vi "DAQmx for CI and AI.vi"() -> (2 "CI Timing Setting":T1={"Sample Clock Source"="PFI0", "Sample Rate"=5.0, "Samples per Loop"=1}, 3 "CI Channel Setting":T2={"Counter"="Dev1/ctr0", "A Input Terminal"="PFI8", "B Input Terminal"="PFI10", "Pulses Per Revolution"=24, "Z Index Enable"=FALSE, "Z Index Terminal"="PFI9"})   [LabVIEW 2017]
panel:
  in  "Timing Setting":T1={"Sample Clock Source"="PFI0", "Sample Rate"=5.0, "Samples per Loop"=1}
  in  "Channel Setting":T2={"Counter"="Dev1/ctr0", "A Input Terminal"="PFI8", "B Input Terminal"="PFI10", "Pulses Per Revolution"=24, "Z Index Enable"=FALSE, "Z Index Terminal"="PFI9"}
  # "CI"
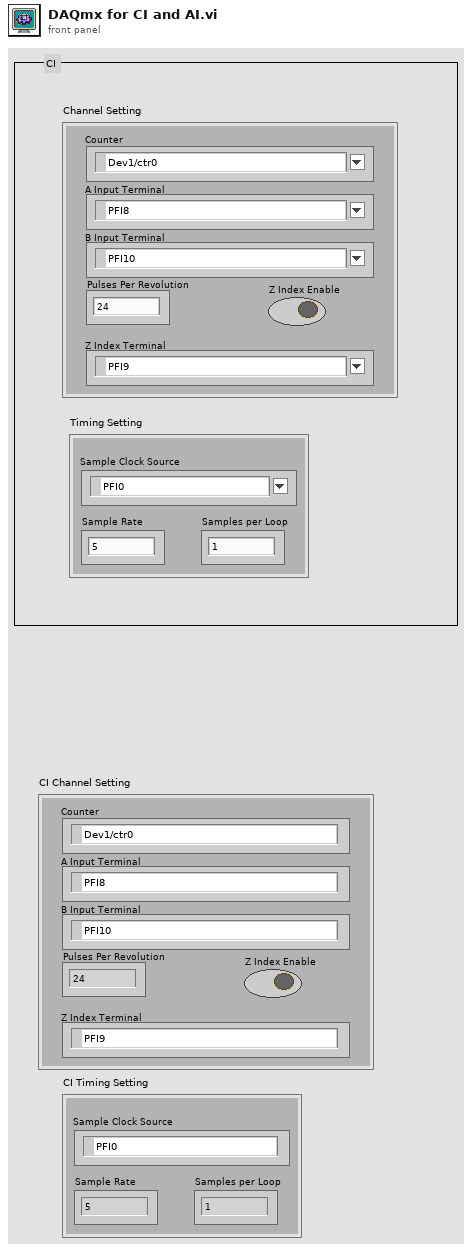
[diagram p1: front panel]
types:
  T1 = cluster{"Sample Clock Source":tag, "Sample Rate":dbl, "Samples per Loop":i32}
  T2 = cluster{"Counter":tag, "A Input Terminal":tag, "B Input Terminal":tag, "Pulses Per Revolution":u32, "Z Index Enable":bool, "Z Index Terminal":tag}
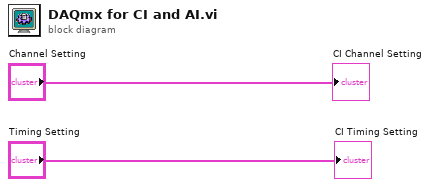
[diagram p0: block diagram]
diagram:
  "CI Channel Setting" <- "Channel Setting"
  "CI Timing Setting" <- "Timing Setting"
